vi "DAQ_E_mIO_DIO.set bit.vi"(0 "i ref in":refnum<vi>, 1 "bit":bool, 2 "bitNo":u32, 3 "ms timeout (10000)":i32=10000, 5 "error in (no error)":errorcluster) -> (14 "i ref out":refnum<vi>, 17 "timed out":bool, 19 "error out":errorcluster)   [LabVIEW 2014, in "DAQ_E_mIO_DIO.lvlib"]
doc: "Sets a bit on a digital output port.\n\nLicense Agreement for this software:\n\nCopyright (C)\nGesellschaft für Schwerionenforschung, GSI\nPlanckstr. 1\n64291 Darmstadt\nGermany\n\nContact: D.Beck@gsi.de \n\nThis program is free software; you can redistribute it and/or modify it under the terms of the GNU General Public License as published by the Free Software Foundation; either version 2 of the license, or (at your option) any later version.\n\nThis program is distributed in the hope that it will be useful, but WITHOUT ANY WARRANTY; without even the implied warranty of MERCHANTABILITY or FITNESS FOR A PARTICULAR PURPOSE. See the GNU General License for more details (http://www.gnu.org).\n\nGesellschaft für Schwerionenforschung, GSI\nPlanckstr. 1, 64291 Darmstadt, Germany\nFor all questions and ideas contact: M.Richter@gsi.de, H.Brand@gsi.de or D.Beck@gsi.de.\nLast update: 17-JUN-2004"
uses:
  DAQ_E_mIO_DIO.lvlib
  CSCore/CSSystem/CoreDefs/CoreDefs.error_type.ctl
  CSApplicationBaseClasses/DigiIOBase/DigiIOBase.directionType.ctl
  CSApplicationBaseClasses/DigiIOBase/DigiIOBase.serviceType.ctl
  lib.lib/UtilityLib/UtilityLib.valueStatus.ctl
  <vilib>/DAQmx/write.llb/DAQmx Write (Digital 1D Bool 1Chan 1Samp).vi
  CSCore/CSSystem/CoreLib/CoreLib.lvlib
  CSApplicationBaseClasses/DigiIOBase/DigiIOBase.lvlib
  lib.lib/UtilityLib/UtilityLib.lvlib
  <resource>/objmgr/daqmx.rc
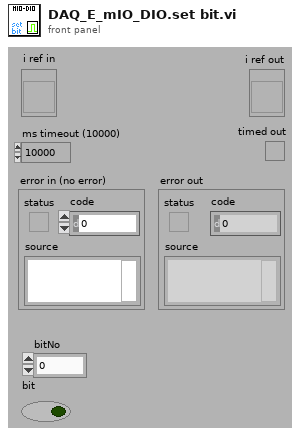
[diagram p1: front panel]
types:
  T1 = typedef "CoreDefs.error_type.ctl" = enum16{"no error", "can't load process", "can't unload process", "process does not exist", "can't install process", "can't remove process", "unknown function", "time out", "can't execute function", "duplicate queue name", "super not found", "caller queue invalid", "can't ping process", "unknown error", "VISA Error", "VISA timeout", "GPIB timeout", "GPIB error", "communication error", "data type mismatch", "can't read data from OPC server", "can't write data to OPC server", "OET error", "function not implemented", "process already exists", "invalid Shared Variable name", "error writing Shared Variable", "error reading Shared Variable", "invalid client name", "corrupt database", "unknown class", "call not authorized", "parameter out of range", "OET timeout: can't get data to modify", "invalid queue name", "requested operation incompatible with current state", "event undefined", "event disabled", "state undefined", "caller is not a friend", "EventBuilder: bad eventID", "EventBuilder: no DAQ devices", "a thread must not stop itself", "UNUSED ELEMENT4", "DiscArchiver: eventData incomplete", "DiscArchiver: eventData does not belong to run", "DiscArchiver: can't open file", "DiscArchiver: can't write to file", "DiscArchiver: available disc space low", "can't acquire semaphore", "error reading data from database", "notifier object is not existing", "can't register process", "can't unregister process", "illegal event type", "object disabled", "object already exists", "can't change state", "Instrument not found", "no connection to remote node", "invalid reference", "N/A", "UNUSED ELEMENT 1", "element not found", "illegal TCP/IP connection detected", "object does not exist", "invalid access ID", "unknown CS system", "invalid privilige", "unsupported data type", "unsupported server type", "IO server already exists", "Shared Variable already exists"}
  T2 = typedef "UtilityLib.lvlib/UtilityLib.valueStatus.ctl" = enum16{"no info available", "stand by/off", "on", "warning", "alarm/malfunction", "not implemented", "user action required", "important information", "system default", "control default", "indicator default", "button default"}
  T3 = typedef "DigiIOBase.lvlib/DigiIOBase.serviceType.ctl" = enum16{"bit", "word"}
  T4 = typedef "DigiIOBase.lvlib/DigiIOBase.directionType.ctl" = enum16{"unknown", "update actual value", "update nominal value", "update both"}
  T5 = typedef "DAQ_E_mIO_DIO.lvlib/DAQ_E_mIO_DIO.i attribute.ctl" = cluster{"DOutChannel":refnum<k21>, "DInChannel":refnum<k21>, "nOfBitsIn":i32, "nOfBitsOut":i32}
  T6 = typedef "DigiIOBase.lvlib/DigiIOBase.i attribute.ctl" = cluster{"logicalName":string[], "physicalName":string[], "logicalNameID":i32, "physicalNameID":i32, "nofBits":i32, "nofBitsID":i32, "nofWords":i32, "nofWordsID":i32, "nomValues":T7, "actValues":T7}
  T7 = typedef "DigiIOBase.lvlib/DigiIOBase.parameters.ctl" = cluster{"high":bool[], "serviceIDs":cluster{"highID":i32}}
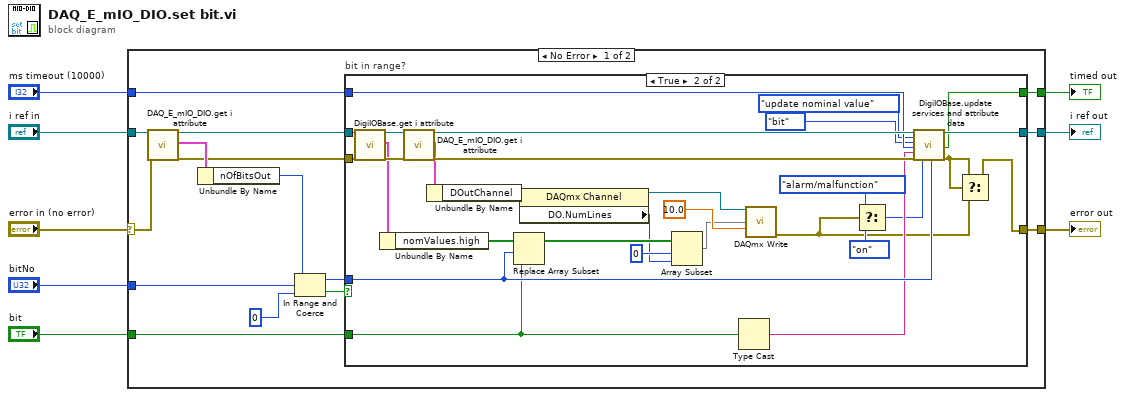
[diagram p0: block diagram]
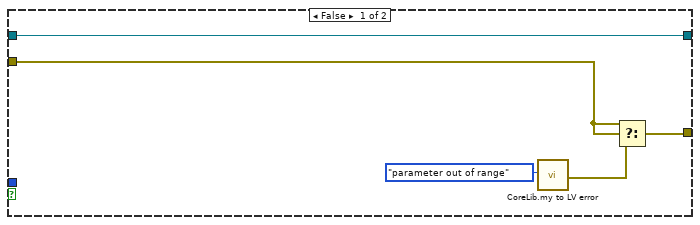
[diagram p2: hidden frame]
diagram:
  n1 = case shown="No Error" "error in (no error)" {
    selector: "error in (no error)" -> [w11 w59]
    tunnel: "i ref in" -> [w19 w60]
    tunnel: "ms timeout (10000)" -> [w23 _]
    tunnel: [w9 _] -> w6
    tunnel: [w22 w60] -> w5
    tunnel: [w21 w59] -> w4
    tunnel: "bitNo" -> [w18 _]
    tunnel: "bit" -> [w20 _]
    frame No Error {
      n2 = call "DAQ_E_mIO_DIO.get i attribute.vi"("i ref in"=w19, "error in (no error)"=w11) -> ("i ref out"=w12:refnum<vi>, "i attribute"=w16:T5, "error out"=w10:errorcluster)  [unwired: 15 in]
      n3 = Unbundle By Name(w16) -> ("nOfBitsOut"=w15:i32)
      n4 = In Range and Coerce(upper limit=w15, x=w18, lower limit=u32 0) -> (coerced(x)=w13:u32, In Range?=w14:bool)
      n5 = case "bit in range?" shown="True" w14 {
        tunnel: w12 -> [w28 w51]
        tunnel: w10 -> [w27 w50]
        tunnel: w23 -> [_ w45]
        tunnel: [w28 w57] -> w22
        tunnel: [w26 w55] -> w21
        tunnel: w13 -> [_ w42]
        tunnel: w20 -> [_ w41]
        tunnel: [_ w39] -> w9
        frame False {
          n6 = call "CoreLib.my to LV error.vi"("ErrorTypes"=CoreDefs.error_type."parameter out of range") -> ("myErrorCluster"=w25:errorcluster)  [unwired: 17 in, 1 out]
          n7 = Select(t=w27, s=w27, f=w25) -> (s? t:f=w26:errorcluster)
        }
        frame True {
          n8 = call "DigiIOBase.get i attribute.vi"("i ref in"=w51, "error in (no error)"=w50) -> ("i ref out"=w49:refnum<vi>, "i attribute"=w47:T6, "error out"=w48:errorcluster)  [unwired: 15 in]
          n9 = Unbundle By Name(w47) -> ("nomValues.high"=w46:bool[])
          n10 = call "DAQ_E_mIO_DIO.get i attribute.vi"("i ref in"=w49, "error in (no error)"=w48) -> ("i ref out"=w58:refnum<vi>, "i attribute"=w54:T5, "error out"=w56:errorcluster)  [unwired: 15 in]
          n11 = Unbundle By Name(w54) -> ("DOutChannel"=w34:refnum<k21>)
          n12 = Replace Array Subset(array=w46, new element=w41, index=w42) -> (w32:bool[])
          n13 = property class="DAQmx Channel"(reference=w34) -> (reference out=w33:refnum<k21>, "DO.NumLines"=w29:u32)  [unwired: 1 in, 1 out]
          n14 = Array Subset(array=w32, index=0, length=w29) -> (w31:bool[])
          n15 = Type Cast(x=w41) -> (*(type *) &x=w40:string)  [unwired: 1 in]
          n16 = call-poly <vilib>:"DAQmx Write.vi"("task/channels in"=w33, "data"=w31, "timeout"=10.0) -> ("error out"=w35:errorcluster)  [unwired: 10 in, 2 out]
          n17 = Select(t=UtilityLib.valueStatus."alarm/malfunction", s=w35, f=UtilityLib.valueStatus."on" ("quality")) -> (s? t:f=w36:T2)
          n18 = call "DigiIOBase.update services and attribute data.vi"("i ref in"=w58, "direction"=DigiIOBase.directionType."update nominal value", "service"=DigiIOBase.serviceType."bit", "ms timeout (10000)"=w45, "value"=w40, "error in (no error)"=w56, "quality"=w36, "index"=w42) -> ("i ref out"=w57:refnum<vi>, "timed out"=w39:bool, "error out"=w53:errorcluster)  [unwired: 9 in]
          n19 = Select(t=w53, s=w53, f=w35) -> (s? t:f=w55:errorcluster)
        }
      }
    }
    frame Error {
    }
  }
  "error out" <- w4
  "i ref out" <- w5
  "timed out" <- w6
